vi "Compound_Arithmatic.vi"() -> ()   [LabVIEW 2019]
panel:
  out "Multiplication":u16
  out "Addition":u8
  in  "Numeric 4":u8
  in  "Numeric 3":u8
  in  "Numeric 2":u8
  in  "Numeric":u8
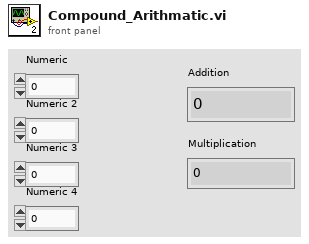
[diagram p1: front panel]
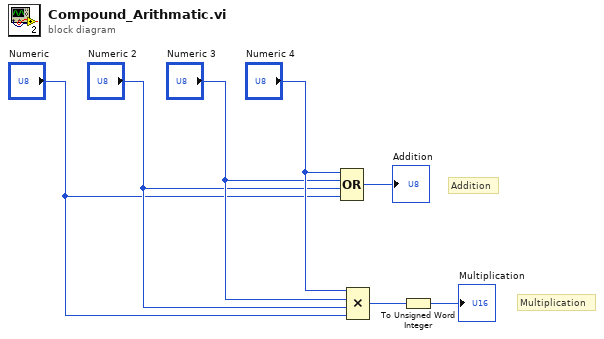
[diagram p0: block diagram]
diagram:
  # "Multiplication"
  # "Addition"
  n1 = Compound Arithmetic op=OR("Numeric 4", "Numeric 3", "Numeric 2", "Numeric") -> (→"Addition":u8)
  n2 = Compound Arithmetic op=MULTIPLY("Numeric 4", "Numeric 3", "Numeric 2", "Numeric") -> (w1:u8)
  n3 = To Unsigned Word Integer(number=w1) -> (unsigned 16bit integer=→"Multiplication":u16)
